vi "Duty Cycle (subVI).vi"(1 "Potentiometer":fxp<+/-,26,5> format="%.23g") -> (0 "Duty Cycle":fxp<+/-,64,12> format="%.56g")   [LabVIEW 2016]
doc: "This subVI supports a PWM output application. It translates a potentiometer reading between 0V and 4V to a duty cycle between 0 and 1."
panel:
  # "This subVI supports a PWM output application.  It translates a potentiometer reading between 0V and 4V to a duty cycle between 0 and 1."
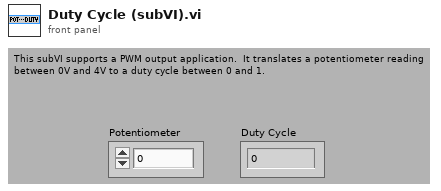
[diagram p1: front panel]
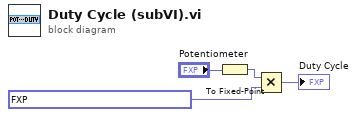
[diagram p0: block diagram]
diagram:
  n1 = To Fixed-Point(number="Potentiometer") -> (fixed-point=w3:fxp<+/-,32,6>)  [unwired: 1 out]
  n2 = Multiply(x=w3, y=fxp<+/-,32,6> 0.25) -> (x*y=→"Duty Cycle":fxp<+/-,64,12>)
